vi "DoaComMusic.vi"() -> ()   [LabVIEW 2018]
uses:
  <vilib>/Analysis/Matrix/Datatypes/ComplexMatrix.ctl
  <vilib>/Analysis/7linalg.llb/Complex Eigenvalues and Vectors.vi
  <vilib>/Analysis/Matrix/Numeric/Multiply/Multiply - CM,CM.vi
  <vilib>/Analysis/Matrix/NI_Matrix.lvlib
  <vilib>/Analysis/NI_AALPro.lvlib
panel:
  out "A * B":T1
  out "Array":cdb[][](array[numeric])
  out "Matrix D":cdb[][](array[numeric])
  in  "Frequência digital (graus)":dbl[][](array[numeric])
  in  "DOA":dbl[][](array[numeric])
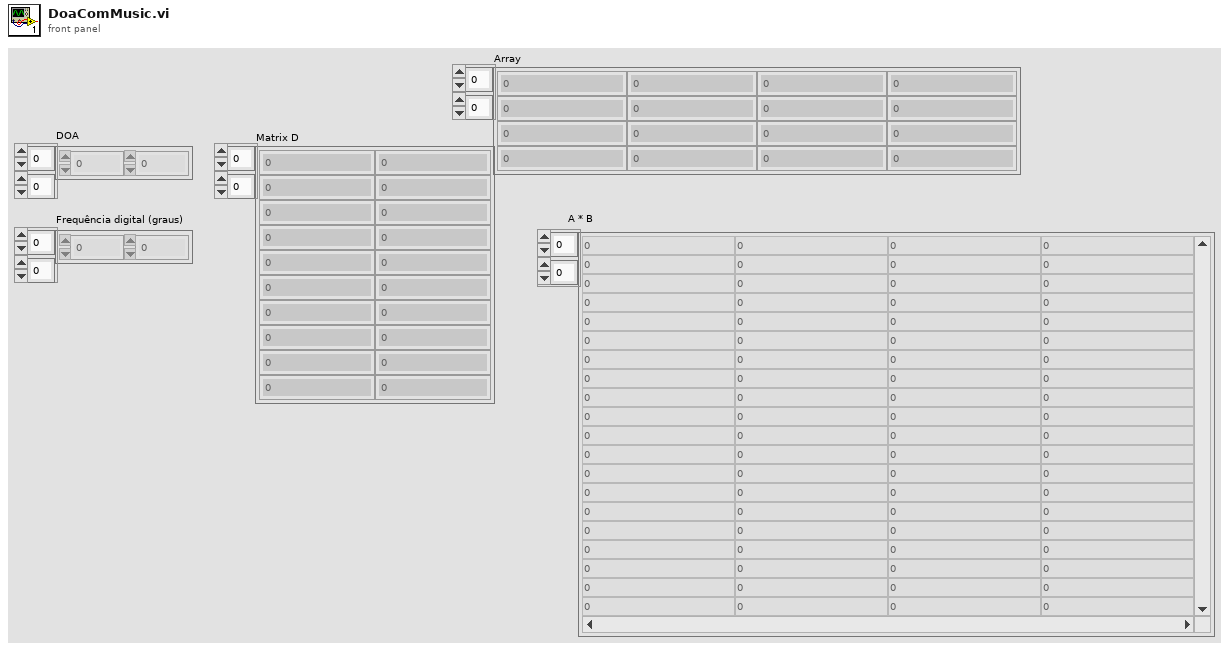
[diagram p1: front panel]
types:
  T1 = typedef "NI_Matrix.lvlib/ComplexMatrix.ctl" = cdb[][]
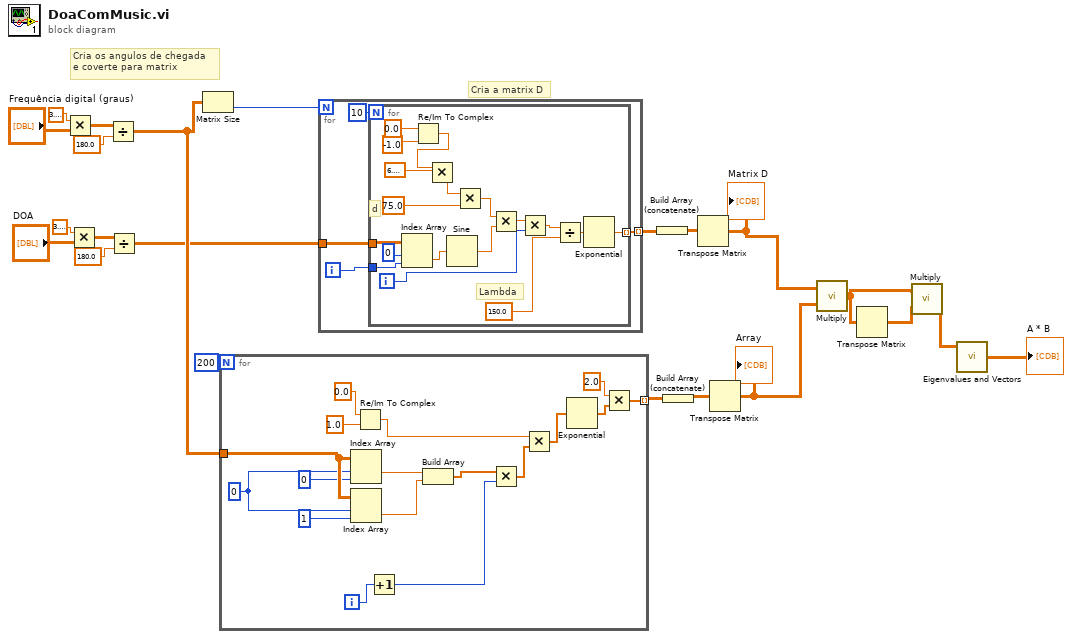
[diagram p0: block diagram]
diagram:
  # "Cria a matrix D"
  # "Cria os angulos de chegada\ne coverte para matrix"
  n1 = Multiply(x=3.141592653589793, y="Frequência digital (graus)") -> (x*y=w19:dbl[][])
  n2 = Multiply(x=3.141592653589793, y="DOA") -> (x*y=w22:dbl[][])
  n3 = Divide(x=w19, y=180.0) -> (x/y=w11:dbl[][])
  n4 = Divide(x=w22, y=180.0) -> (x/y=w10:dbl[][])
  n5 = Matrix Size(0:w11) -> (2:w15:i32)  [unwired: 1 out]
  n6 = for {
    N: 200 -> [_]
    tunnel: w11 -> [w29]
    tunnel: [w30] -> w9 mode=indexing
    i -> [w35]
    w28 = 0 ("index (row)")
    n7 = Index Array(array=w29, index (row)=w28, index (col)=0) -> (element=w25:dbl)
    n8 = Index Array(array=w29, index (row)=w28, index (col)=1) -> (element=w24:dbl)
    n9 = Re/Im To Complex(1:1.0 ("y"), 2:0.0 ("x")) -> (0:w32:cdb)
    n10 = Increment(x=w35) -> (x+1=w34:i32)
    n11 = Build Array(w25, w24) -> (w23:dbl[])
    n12 = Multiply ("Multiply.vi")(x=w23, y=w34) -> (x*y=w33:dbl[])
    n13 = Multiply ("Multiply.vi")(x=w32, y=w33) -> (x*y=w31:cdb[])
    n14 = Exponential ("Exponential.vi")(1:w31) -> (0:w38:cdb[])
    n15 = Multiply ("Multiply.vi")(x=2.0, y=w38) -> (x*y=w30:cdb[])
  }
  n16 = for {
    N: w15 -> [_]
    tunnel: w10 -> [w42]
    tunnel: [w40] -> w13 mode=indexing
    i -> [w41]
    n17 = for {
      N: 10 -> [_]
      tunnel: w42 -> [w57]
      tunnel: w41 -> [w55]
      tunnel: [w47] -> w40 mode=indexing
      i -> [w44]
      # "d"
      # "Lambda"
      n18 = Index Array(array=w57, index (row)=0, index (col)=w55) -> (element=w54:dbl)
      n19 = Re/Im To Complex(1:-1.0 ("y"), 2:0.0 ("x")) -> (0:w59:cdb)
      n20 = Multiply(x=w59, y=6.283185307179586) -> (x*y=w53:cdb)
      n21 = Sine(x=w54) -> (sin(x)=w50:dbl)
      n22 = Multiply(x=w53, y=75.0) -> (x*y=w51:cdb)
      n23 = Multiply(x=w51, y=w50) -> (x*y=w46:cdb)
      n24 = Multiply(x=w46, y=w44) -> (x*y=w45:cdb)
      n25 = Divide(x=w45, y=150.0) -> (x/y=w48:cdb)
      n26 = Exponential(1:w48) -> (0:w47:cdb)
    }
  }
  n27 = Build Array (concatenate)(w13) -> (w12:T1)
  n28 = Build Array (concatenate)(w9) -> (w8:T1)
  n29 = Transpose Matrix(1:w12) -> (0:w7:T1)
  "Matrix D" <- w7
  n30 = Transpose Matrix(1:w8) -> (0:w6:T1)
  "Array" <- w6
  n31 = call-poly <vilib>:"Multiply.vi"("Complex Matrix B"=w6, "Complex Matrix A"=w7) -> ("A * B"=w5:T1)
  n32 = Transpose Matrix(1:w5) -> (0:w4:T1)
  n33 = call-poly <vilib>:"Multiply.vi"("Complex Matrix B"=w4, "Complex Matrix A"=w5) -> ("A * B"=w2:T1)
  n34 = call-poly <vilib>:"Eigenvalues and Vectors.vi"("Input Matrix"=w2) -> ("Eigenvectors"=→"A * B":T1)  [unwired: 2 in, 2 out]
